vi "Test Reg0Write Generate Vector Statements.vi"(10 "Register Data":T1 format="%02x", 11 "Slave Address":T2=12 format="%02x") -> (1 "Vector Statements":string[][](array[string]), 2 "register address equal":bool, 3 "Slave address match":bool)   [LabVIEW 2018, in "MIPI RFFE API.lvlib" / "RFFE Command.lvclass"]
uses:
  Command/RFFE Command.lvclass
  Slave Address.ctl
  Register Data.ctl
  Reg0Write/RFFE Reg0Write Command.lvclass
  MIPI RFFE API.lvlib
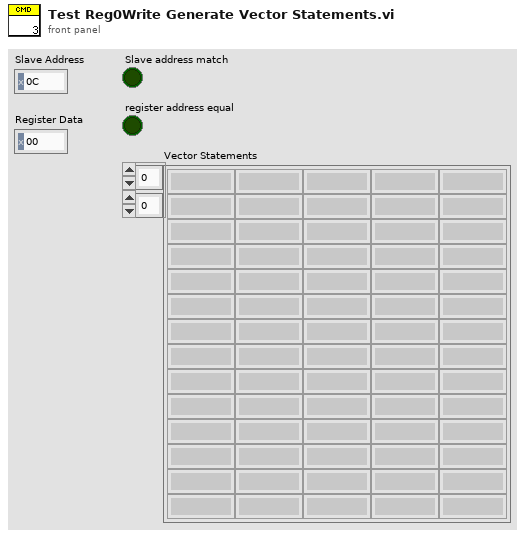
[diagram p1: front panel]
types:
  T1 = typedef "MIPI RFFE API.lvlib/Register Data.ctl" = u8
  T2 = typedef "MIPI RFFE API.lvlib/Slave Address.ctl" = u8
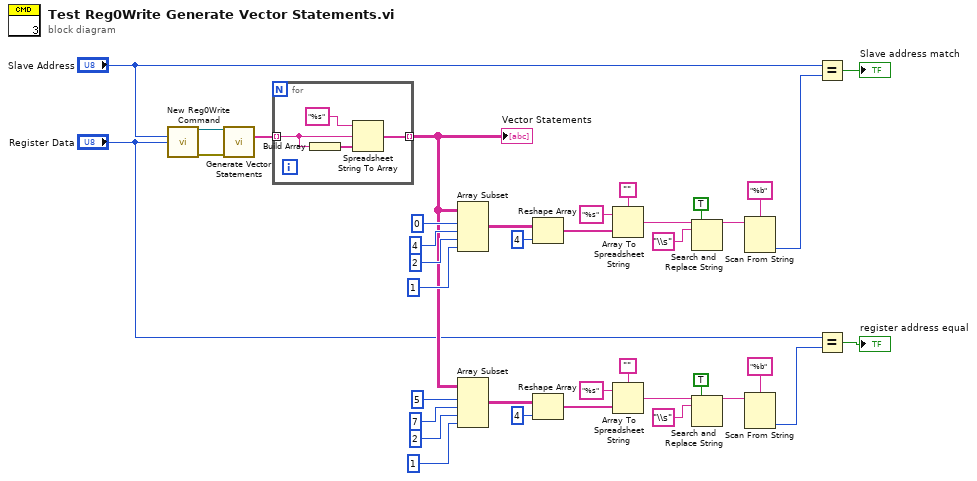
[diagram p0: block diagram]
diagram:
  n1 = call "New Reg0Write Command.vi"("Slave Address"="Slave Address", "Register Data"="Register Data") -> ("RFFE Reg0Write Command out"=w38:refnum<class "RFFE Reg0Write Command.lvclass">, "error out"=w37:errorcluster)  [unwired: 12 in]
  n2 = call-dynamic "Generate Vector Statements.vi"("RFFE Command in"=w38, "error in (no error)"=w37) -> ("Vector Statements"=w36:string[])  [unwired: 11 in, 2 out]
  n3 = for {
    tunnel: w36 -> [w41] mode=indexing
    tunnel: [w39] -> w3 mode=indexing
    n4 = Build Array(w41) -> (w42:string[])
    n5 = Spreadsheet String To Array(format string="%s", spreadsheet string=w41, array type (2D Dbl)=w42) -> (array=w39:string[])  [unwired: 1 in]
  }
  "Vector Statements" <- w3
  n6 = Array Subset(array=w3, index (row)=0 ("index"), length (row)=4 ("length"), index (col)=2 ("index"), length (col)=1 ("length")) -> (w31:string[][])
  n7 = Array Subset(array=w3, index (row)=5 ("index"), length (row)=7 ("length"), index (col)=2 ("index"), length (col)=1 ("length")) -> (w8:string[][])
  n8 = Reshape Array(w31, 4 ("dimension size")) -> (w29:string[])
  n9 = Reshape Array(w8, 4 ("dimension size")) -> (w10:string[])
  n10 = Array To Spreadsheet String(delimiter (Tab)="", array=w29, 3:"%s" ("format string")) -> (spreadsheet string=w24:string)
  n11 = Array To Spreadsheet String(delimiter (Tab)="", array=w10, 3:"%s" ("format string")) -> (spreadsheet string=w15:string)
  n12 = Search and Replace String(replace all?=TRUE ("replace all? (F)"), input string=w24, search string="\\s") -> (result string=w26:string)  [unwired: 5 in, 3 out]
  n13 = Search and Replace String(replace all?=TRUE ("replace all? (F)"), input string=w15, search string="\\s") -> (result string=w13:string)  [unwired: 5 in, 3 out]
  n14 = Scan From String(format string="%b", input string=w26) -> (output 1=w20:i32)  [unwired: 3 in, 3 out]
  n15 = Scan From String(format string="%b", input string=w13) -> (output 1=w2:i32)  [unwired: 3 in, 3 out]
  n16 = Equal?(x="Slave Address", y=w20) -> (x = y?=→"Slave address match":bool)
  n17 = Equal?(x="Register Data", y=w2) -> (x = y?=→"register address equal":bool)
